vi "Untitled5.vi"() -> ()   [LabVIEW 2017]
panel:
  in  "Array 6":string[](array[string])
  in  "Thresholds":u16=600
  in  "one key for threshold":bool
  in  "SMA mode":bool=TRUE
  in  "Thresholds (mV)":u16[](array[numeric])
  out "Array":u32[](array[numeric])=[96, 98, 100, 102, 104, 106, 108, 110, 128, 130, 132, 134, 136, 138, 140, 142, 160, 162, 164, 166, 168, 170, 172, 174, 192, 194, 196, 198, 200, 202, 204, 206] format="%x"
  out "Array 2":u32[](array[numeric])=[97, 99, 101, 103, 105, 107, 109, 111, 129, 131, 133, 135, 137, 139, 141, 143, 161, 163, 165, 167, 169, 171, 173, 175, 193, 195, 197, 199, 201, 203, 205, 207] format="%x"
  out "Array 3":u32[](array[numeric])=[0, 0, 0, 0, 0, 0, 0, 0, 32, 32, 32, 32, 32, 32, 32, 32, 64, 64, 64, 64, 64, 64, 64, 64, 96, 96, 96, 96, 96, 96, 96, 96] format="%x"
  out "Array 4":u32[](array[numeric])=[96, 96, 96, 96, 96, 96, 96, 96, 128, 128, 128, 128, 128, 128, 128, 128, 160, 160, 160, 160, 160, 160, 160, 160, 192, 192, 192, 192, 192, 192, 192, 192] format="%x"
  out "Array 5":u32[](array[numeric])=[0, 2, 4, 6, 8, 10, 12, 14, 0, 2, 4, 6, 8, 10, 12, 14, 0, 2, 4, 6, 8, 10, 12, 14, 0, 2, 4, 6, 8, 10, 12, 14] format="%x"
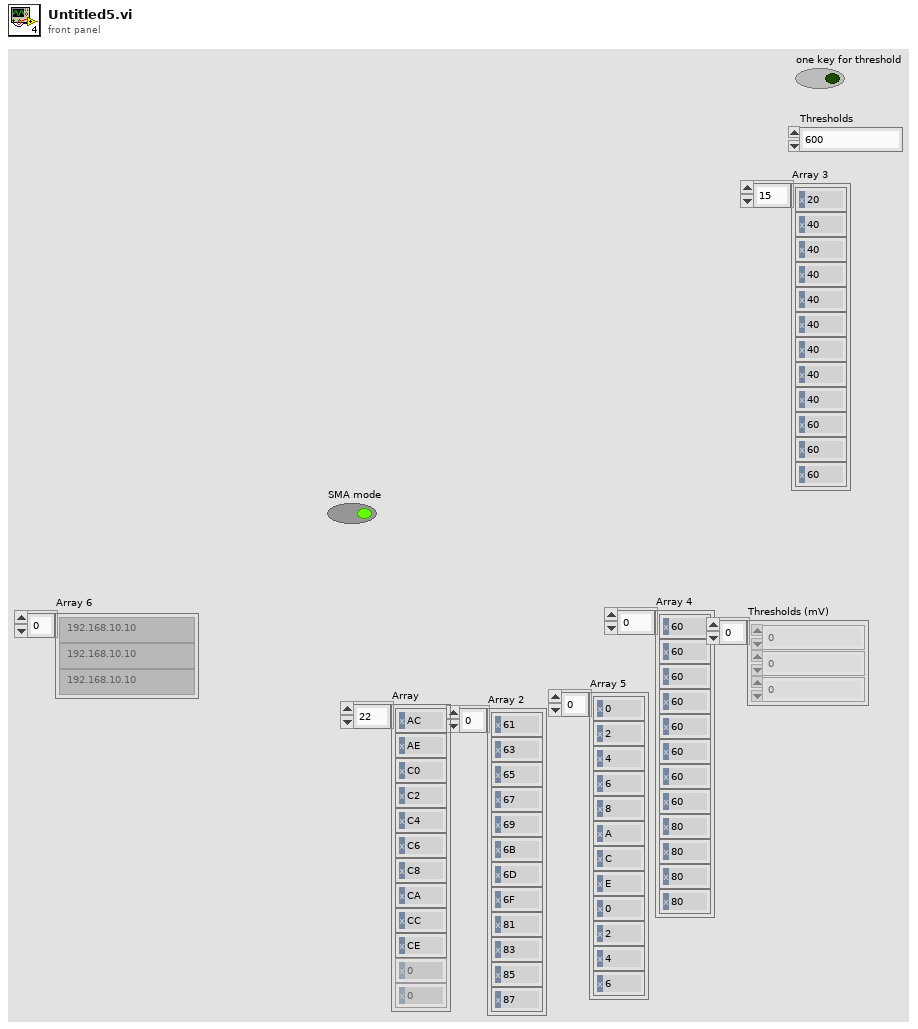
[diagram p1: front panel]
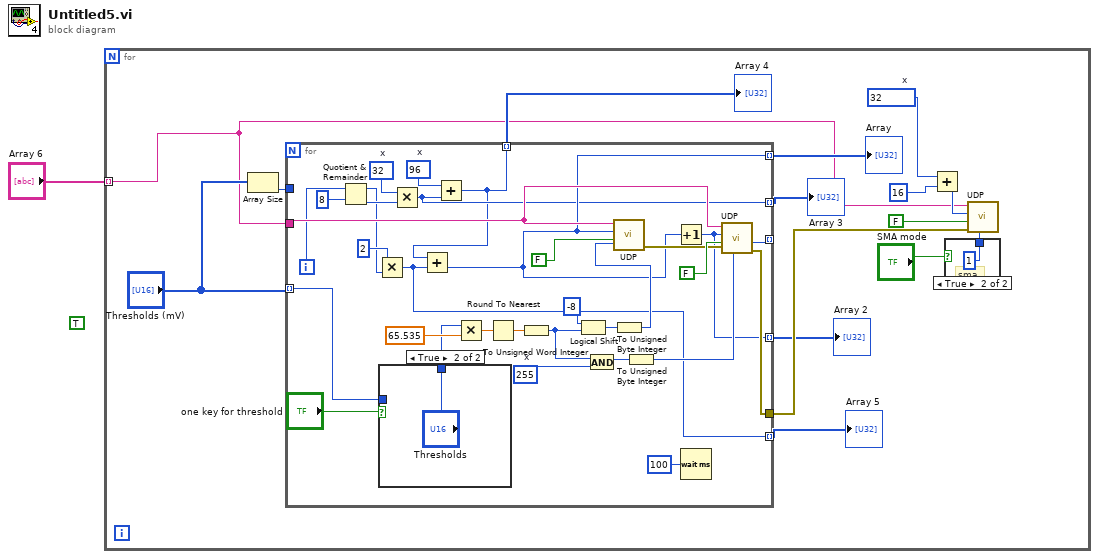
[diagram p0: block diagram]
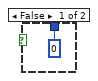
[diagram p2: hidden frame]
diagram:
  (unwired) TRUE
  n1 = for {
    tunnel: "Array 6" -> [w2] mode=indexing
    w4 = u16 32  # x
    n2 = Array Size(array="Thresholds (mV)") -> (size(s)=w12:i32)
    n3 = for {
      tunnel: w2 -> [w45]
      tunnel: "Thresholds (mV)" -> [w31] mode=indexing
      tunnel: [w39] -> _ mode=indexing
      tunnel: [w34] -> w15
      tunnel: w12 -> [_]
      tunnel: [w25] -> w10 mode=indexing
      tunnel: [w24] -> w9 mode=indexing
      tunnel: [w23] -> w8 mode=indexing
      tunnel: [w22] -> w7 mode=indexing
      tunnel: [w21] -> w6 mode=indexing
      i -> [w26]
      w27 = u16 96  # x
      w28 = u16 32  # x
      w41 = u16 255  # x
      n4 = Quotient & Remainder(x=w26, y=8) -> (x-y*floor(x/y)=w20:i32, floor(x/y)=w29:i32)
      n5 = Multiply(x=2, y=w20) -> (x*y=w21:i32)
      n6 = case shown="True" "one key for threshold" {
        tunnel: [w51 "Thresholds"] -> w32
        tunnel: w31 -> [w51 _]
        frame False {
        }
        frame True {
        }
      }
      n7 = Multiply(x=w28, y=w29) -> (x*y=w23:i32)
      n8 = Add(x=w27, y=w23) -> (x+y=w22:i32)
      n9 = Add(x=w22, y=w21) -> (x+y=w25:i32)
      n10 = Multiply(x=w32, y=65.535) -> (x*y=w48:dbl)
      n11 = Round To Nearest(number=w48) -> (nearest integer value=w46:dbl)
      n12 = To Unsigned Word Integer(number=w46) -> (unsigned 16bit integer=w36:u16)
      n13 = Logical Shift(y=i16 -8, x=w36) -> (x << y=w43:u16)
      n14 = And(x=w36, y=w41) -> (x .and. y?=w40:u16)
      n15 = To Unsigned Byte Integer(number=w43) -> (unsigned 8bit integer=w42:u8)
      n16 = call "UDP.vi"("In"=w42, "Read (TRUE)"=FALSE, "Address"=w25, "IP address"=w45) -> ("error out"=w35:errorcluster)  [unwired: 5 in, 1 out]
      n17 = To Unsigned Byte Integer(number=w40) -> (unsigned 8bit integer=w38:u8)
      n18 = Increment(x=w25) -> (x+1=w24:i32)
      n19 = Wait (ms)(milliseconds to wait=u32 100) -> ()  [unwired: 1 out]
      n20 = call "UDP.vi"("In"=w38, "error in (no error)"=w35, "Read (TRUE)"=FALSE, "Address"=w24, "IP address"=w45) -> ("error out"=w34:errorcluster, "Out"=w39:u8)  [unwired: 4 in]
    }
    "Array" <- w10
    "Array 2" <- w9
    "Array 3" <- w8
    "Array 4" <- w7
    "Array 5" <- w6
    n21 = Add(x=w4, y=u32 16 ("Address")) -> (x+y=w3:u32)
    n22 = case shown="True" "SMA mode" {
      tunnel: [u8 0 ("In") u8 1 ("In")] -> w14
      frame False {
      }
      frame True {
        # "sma"
      }
    }
    n23 = call "UDP.vi"("In"=w14, "error in (no error)"=w15, "Read (TRUE)"=FALSE, "Address"=w3, "IP address"=w2) -> ()  [unwired: 4 in, 2 out]
  }
